vi "Desktop Main.vi"() -> ()   [LabVIEW 2021]
doc: "Demonstrates the use of the Network Streams functions to send LED status to the myRIO target."
uses:
  <vilib>/ErrorRing/Error Ring.xnode
panel:
  in  "Stop":bool
  out "Tank":dbl(slide) scale=0.0..10.0
  out "error out":errorcluster
  in  "Target IP Address":string="172.22.11.2"
  # "Overview: Demonstrates the use of the Network Streams functions to send LED status to the myRIO target.\nInstructions:\n1. Verify the value of Target IP Address. If it is incorrect, specify the correct value.\n2. Run this VI.\n3. Open RT Main.vi and follow its front panel instructions.\n4. Click Stop to stop this VI. Stopping this VI also terminates the running of RT Main.vi."
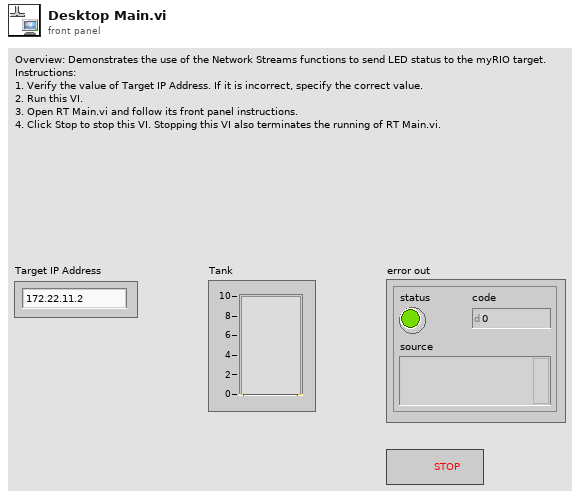
[diagram p1: front panel]
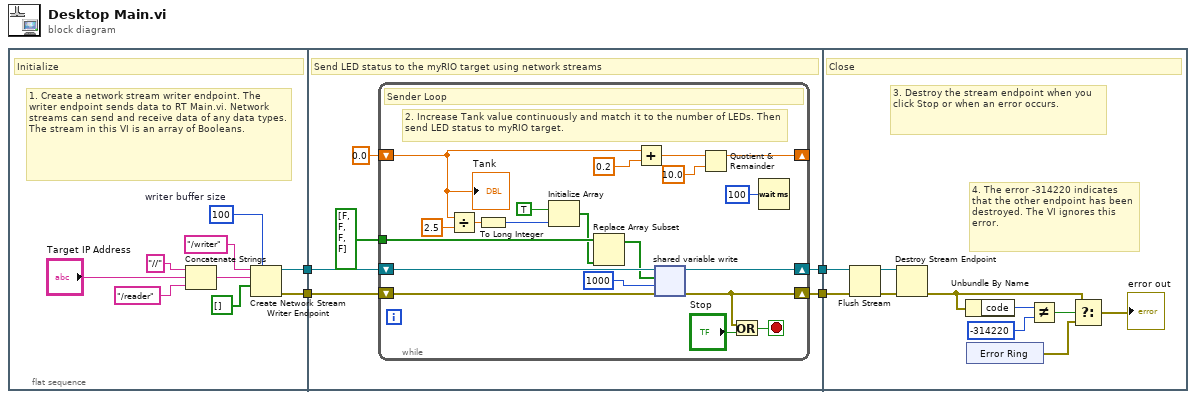
[diagram p0: block diagram]
diagram:
  n1 = flat-sequence {
    tunnel: [w8] -> w4
    tunnel: [w7] -> w1
    tunnel: [w17] -> w3
    tunnel: w4 -> [w19]
    tunnel: [w16] -> w2
    tunnel: w1 -> [w18]
    tunnel: w3 -> [w49]
    tunnel: w2 -> [w46]
    frame #0 {
      w5 = 100  # writer buffer size
      # "1. Create a network stream writer endpoint. The writer endpoint sends data to RT Main.vi. Network streams can send and receive data of any data types. The stream in this VI is an array of Booleans."
      # "Initialize"
      n2 = Concatenate Strings("//", "Target IP Address", "/reader") -> (w13:string)
      n3 = Create Network Stream Writer Endpoint(7:w5, 9:bool[] [], 10:w13, 11:"/writer" ("reader name")) -> (0:w7:errorcluster, 3:w8:refnum<k21>)  [unwired: 3 in]
    }
    frame #1 {
      # "Send LED status to the myRIO target using network streams"
      n4 = while {
        shift-right: [w28] -> w16
        shift-left: w18 -> [w26]
        shift-right: [w29] -> w17
        shift-left: w19 -> [w25]
        shift-right: [w30] -> _
        shift-left: 0.0 -> [w35]
        tunnel: bool[] [FALSE, FALSE, FALSE, FALSE] -> [w22]
        stop <- w39 stop-if-true
        # "2. Increase Tank value continuously and match it to the number of LEDs. Then send LED status to myRIO target."
        # "Sender Loop"
        n5 = Divide(x=w35, y=2.5) -> (x/y=w37:dbl)
        n6 = To Long Integer(number=w37) -> (32bit integer=w24:i32)
        n7 = Initialize Array(TRUE, w24) -> (w21:bool[])
        n8 = Replace Array Subset(array=w22, new element=w21) -> (w20:bool[])  [unwired: 1 in]
        n9 = Add(x=w35, y=0.2) -> (x+y=w31:dbl)
        n10 = shared-variable-write(w25, w26, w20, 1000 ("timeout ms (-1)")) -> (w29:refnum<k21>, w28:errorcluster)  [unwired: 1 out]
        n11 = Quotient & Remainder(x=w31, y=10.0) -> (x-y*floor(x/y)=w30:dbl)  [unwired: 1 out]
        n12 = Or(x=w28, y="Stop") -> (x .or. y?=w39:bool)
        n13 = Wait (ms)(milliseconds to wait=u32 100) -> ()  [unwired: 1 out]
        "Tank" <- w35
      }
    }
    frame #2 {
      # "4. The error -314220 indicates that the other endpoint has been destroyed. The VI ignores this error."
      # "3. Destroy the stream endpoint when you click Stop or when an error occurs."
      # "Close"
      n14 = Flush Stream(8:w46, 11:w49) -> (0:w47:errorcluster, 3:w48:refnum<k21>)  [unwired: 2 in, 1 out]
      n15 = Destroy Stream Endpoint(8:w47, 11:w48) -> (0:w41:errorcluster)
      n16 = Unbundle By Name(w41) -> ("code"=w45:i32)
      n17 = xnode "Error Ring"() -> ("error out"=w42:errorcluster)
      n18 = Not Equal?(x=w45, y=-314220) -> (x != y?=w43:bool)
      n19 = Select(t=w41, s=w43, f=w42) -> (s? t:f=→"error out":errorcluster)
    }
  }
